vi "FCS.vi"(10 "发送命令":string) -> (0 "FCS校验":string, 2 "完整帧":string)   [LabVIEW 2012]
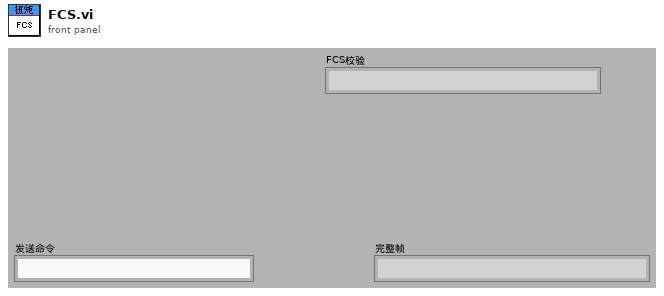
[diagram p1: front panel]
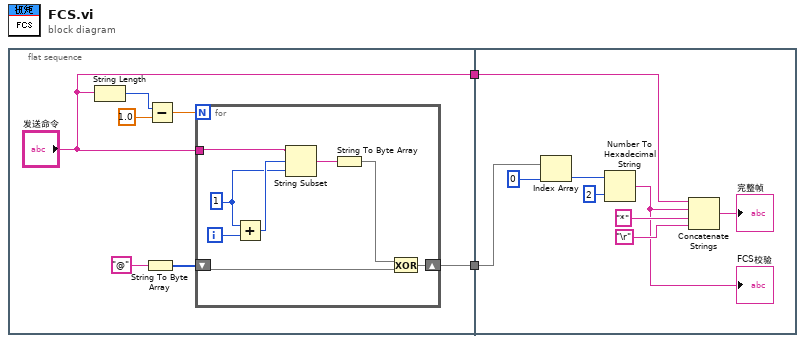
[diagram p0: block diagram]
diagram:
  n1 = flat-sequence {
    tunnel: ["发送命令"] -> w2
    tunnel: [w3] -> w1
    tunnel: w2 -> [w20]
    tunnel: w1 -> [w19]
    frame #0 {
      n2 = String Length(string="发送命令") -> (length=w7:i32)
      n3 = String To Byte Array(string="@") -> (unsigned byte array=w5:u8[])
      n4 = Subtract(x=w7, y=1.0) -> (x-y=w9:dbl)
      n5 = for {
        N: w9 -> [_]
        tunnel: "发送命令" -> [w14]
        shift-right: [w12] -> w3
        shift-left: w5 -> [w10]
        i -> [w16]
        w15 = 1
        n6 = Add(x=w15, y=w16) -> (x+y=w17:i32)
        n7 = String Subset(string=w14, offset (0)=w17, length (rest)=w15) -> (substring=w13:string)
        n8 = String To Byte Array(string=w13) -> (unsigned byte array=w11:u8[])
        n9 = Exclusive Or(1:w10, 2:w11) -> (0:w12:u8[])
      }
    }
    frame #1 {
      n10 = Index Array(array=w19, index=0 ("索引")) -> (element=w25:u8)
      n11 = Number To Hexadecimal String(1:i16 2 ("宽度(-)"), 2:w25) -> (0:w18:string)
      "FCS校验" <- w18
      n12 = Concatenate Strings(w20, w18, "*", "\r") -> (→"完整帧":string)
    }
  }
